vi "IsEven.vi"(1 "Numeric":dbl) -> (0 "Boolean":bool)   [LabVIEW 2013]
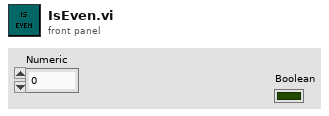
[diagram p1: front panel]
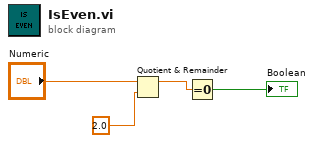
[diagram p0: block diagram]
diagram:
  n1 = Quotient & Remainder(x="Numeric", y=2.0) -> (x-y*floor(x/y)=w2:dbl)  [unwired: 1 out]
  n2 = Equal To 0?(x=w2) -> (x = 0?=→"Boolean":bool)
